vi "Remove Module from Tree.vi"(10 "Node To Remove":string="\\CML 2019.lvproj\\Acquisition.lvlib", 11 "Tree Map Input":T1(c390)) -> (3 "Tree Map Out":T1(c390))   [LabVIEW 2019, in "Panther Dashboard.lvlib"]
uses:
  Panther Dashboard.lvlib
  <vilib>/National Instruments/Tree Map/Tree Map.lvlib
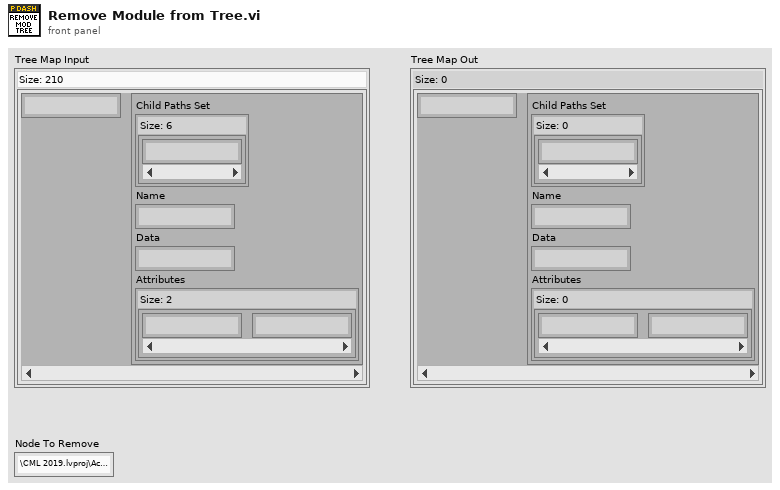
[diagram p1: front panel]
types:
  T1 = map{string, cluster{"Child Paths Set":set{string}, "Name":string, "Data":string, "Attributes":map{string, string}}}
  T2 = typedef "Tree Map.lvlib/Tree Map Data.ctl" = map{string, cluster{"Child Paths Set":set{string}, "Name":string, "Data":string, "Attributes":map{string, string}}}
  T3 = cluster{"Tree Path":string, "Node":cluster{"Child Paths Set":set{string}, "Name":string, "Data":string, "Attributes":map{string, string}}}
  T4 = cluster{"Child Paths Set":set{string}, "Name":string, "Data":string, "Attributes":map{string, string}}
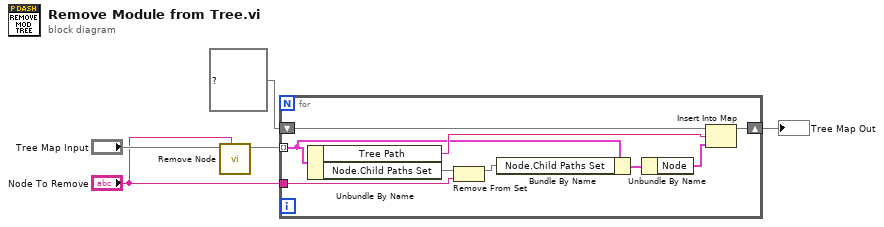
[diagram p0: block diagram]
diagram:
  n1 = call <vilib>:"Remove Node.vi"("Node Path"="Node To Remove", "Tree Map In"="Tree Map Input") -> ("Tree Map Out"=w2:T2)  [unwired: 7 in, 2 out]
  n2 = for {
    tunnel: w2 -> [w11] mode=indexing
    tunnel: "Node To Remove" -> [w14]
    shift-right: [w7] -> w1
    shift-left: T1 {} ("Tree Map Out") -> [w13]
    n3 = Unbundle By Name(w11) -> ("Tree Path"=w12:string, "Node.Child Paths Set"=w6:set{string})
    n4 = Remove From Set(10:w14, 11:w6) -> (3:w10:set{string})  [unwired: 1 out]
    n5 = Bundle By Name(cluster=w11, "Node.Child Paths Set"=w10) -> (w9:T3)
    n6 = Unbundle By Name(w9) -> ("Node"=w8:T4)
    n7 = Insert Into Map(map in=w13, key=w12, value=w8) -> (map out=w7:T1)  [unwired: 2 out]
  }
  "Tree Map Out" <- w1
